vi "extractReIm.vi"(7 "Points":i32, 11 "Input":dbl[](array[numeric])) -> (2 "Im":dbl[](array[numeric]), 3 "Re":dbl[](array[numeric]))   [LabVIEW 2021]
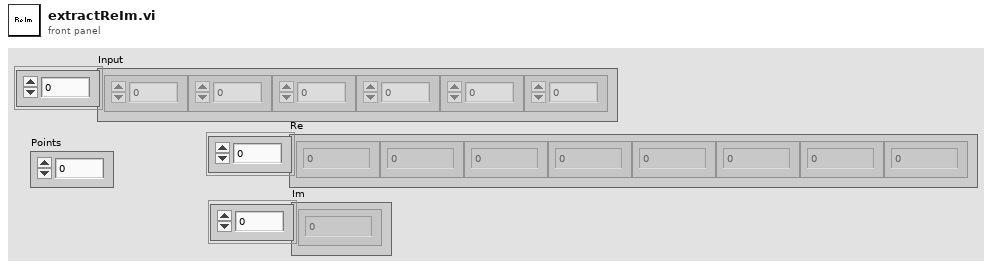
[diagram p1: front panel]
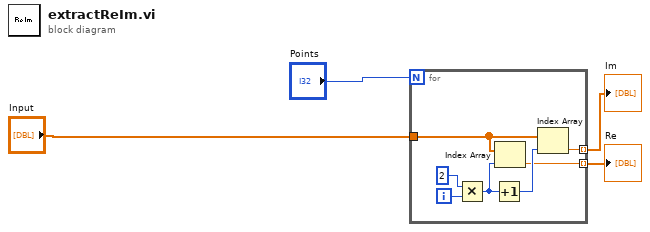
[diagram p0: block diagram]
diagram:
  n1 = for {
    N: "Points" -> [_]
    tunnel: "Input" -> [w11]
    tunnel: [w6] -> w3 mode=indexing
    tunnel: [w5] -> w2 mode=indexing
    i -> [w10]
    n2 = Multiply(x=2, y=w10) -> (x*y=w7:i32)
    n3 = Increment(x=w7) -> (x+1=w8:i32)
    n4 = Index Array(array=w11, index=w7) -> (element=w6:dbl)
    n5 = Index Array(array=w11, index=w8) -> (element=w5:dbl)
  }
  "Re" <- w3
  "Im" <- w2
